vi "编辑控件.vi"(11 "控件类型":string) -> ()   [LabVIEW 2018]
panel:
  in  "图片路径":path
  in  "修改":bool
  in  "删除":bool
  in  "增加":bool
  in  "控件列表":i32(listbox)
  out "图片预览":picture
  in  "程序文本":string
  in  "关键字":string
  in  "控件名称":string
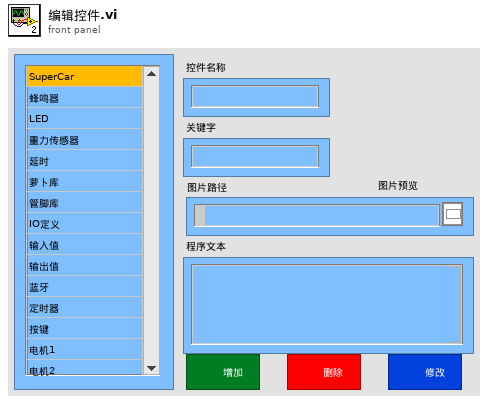
[diagram p1: front panel]
types:
  T1 = typedef "imagedata.ctl" = cluster{"image type":i32, "image depth":i32, "image":u8[], "mask":u8[], "colors":u32[], "Rectangle":cluster{"left":i16, "top":i16, "right":i16, "bottom":i16}}
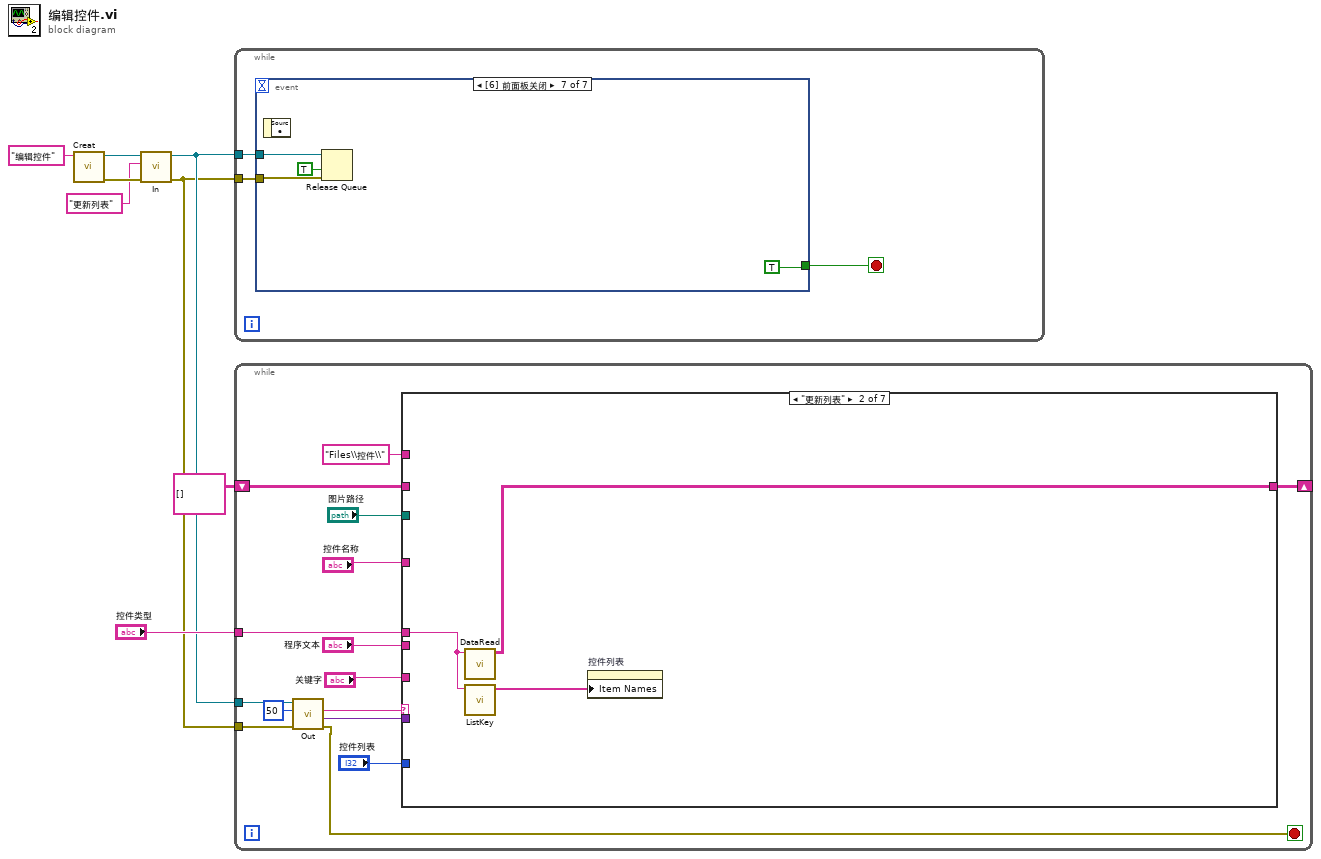
[diagram p0: block diagram]
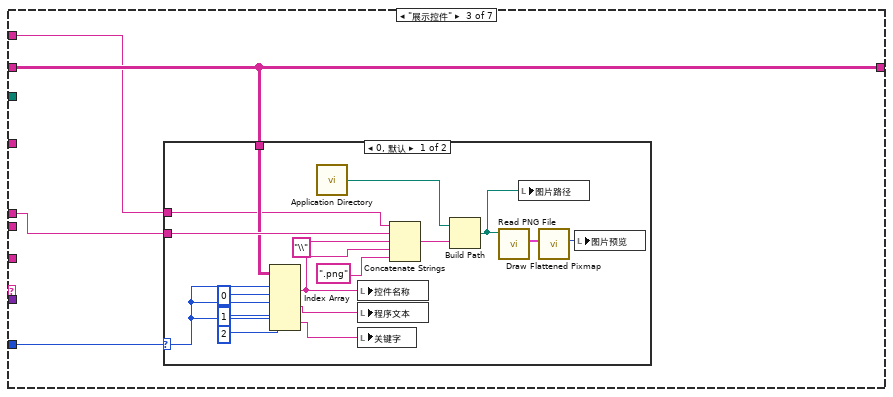
[diagram p3: hidden frame]
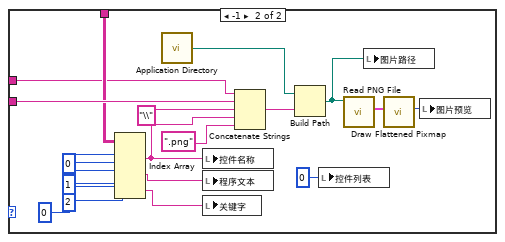
[diagram p4: hidden frame]
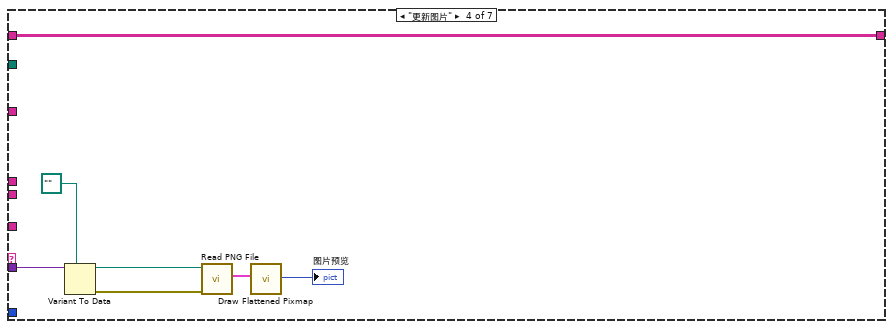
[diagram p5: hidden frame]
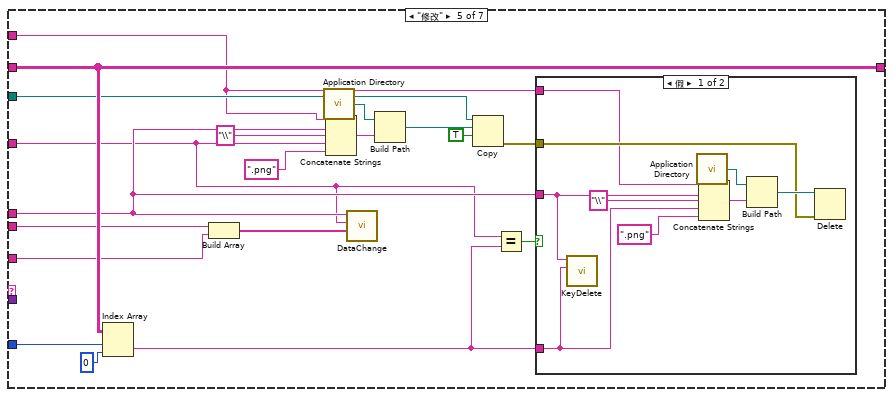
[diagram p6: hidden frame]
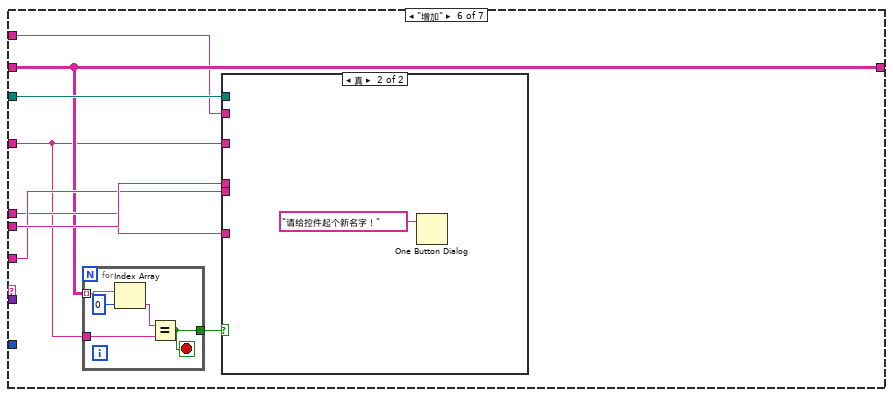
[diagram p8: hidden frame]
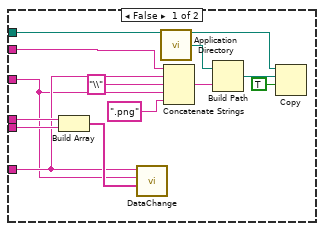
[diagram p9: hidden frame]
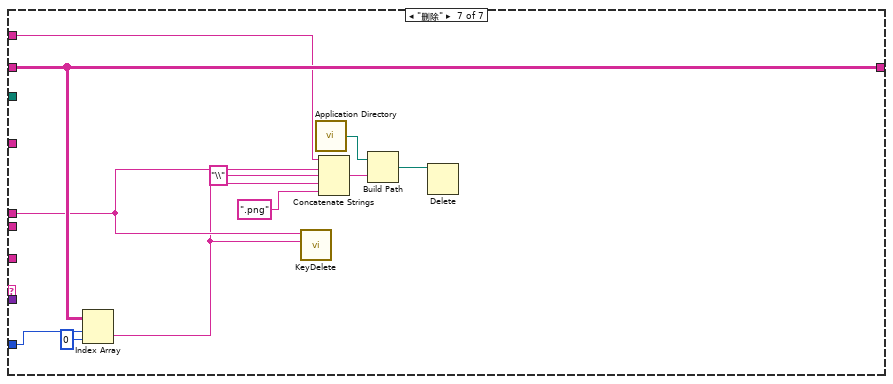
[diagram p10: hidden frame]
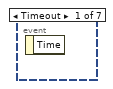
[diagram p11: hidden frame]
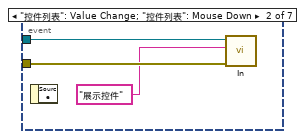
[diagram p12: hidden frame]
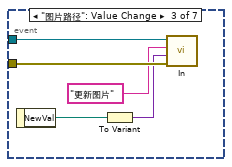
[diagram p13: hidden frame]
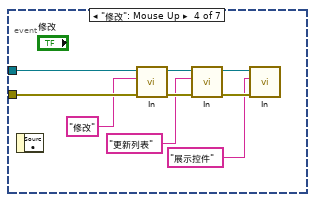
[diagram p14: hidden frame]
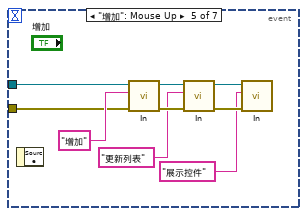
[diagram p15: hidden frame]
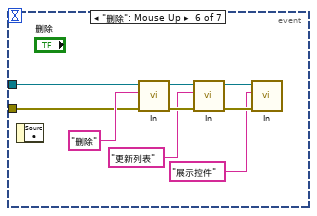
[diagram p16: hidden frame]
diagram:
  n1 = call "Creat.vi"("名称"="编辑控件") -> ("错误输出"=w2:errorcluster, "队列输出"=w5:refnum<queue>)  [unwired: 9 in]
  n2 = call "In.vi"("错误输入"=w2, "指令"="更新列表", "队列"=w5) -> ("错误输出"=w3:errorcluster, "队列输出"=w4:refnum<queue>)  [unwired: 7 in]
  n3 = while {
    tunnel: w4 -> [w11]
    tunnel: w3 -> [w10]
    stop <- w9 stop-if-true
    n4 = event shown="[6] 前面板关闭" {
      selector: _ -> [_ _ _ _ _ _ _]
      dyn-events: _ -> [_ _ _ _ _ _ _]
      timeout: _ -> [_ _ _ _ _ _ _]
      tunnel: w11 -> [_ w14 w19 w28 w30 w39 w49]
      tunnel: w10 -> [_ w13 w18 w27 w29 w38 w48]
      tunnel: [_ _ _ _ _ _ TRUE] -> w9
      event Timeout {
        n5 = event-data() -> ()  [unwired: 1 in, 1 out]
      }
      event "控件列表": Value Change; "控件列表": Mouse Down {
        n6 = event-data() -> ()  [unwired: 1 in, 1 out]
        n7 = call "In.vi"("错误输入"=w13, "指令"="展示控件", "队列"=w14) -> ()  [unwired: 7 in, 2 out]
      }
      event "图片路径": Value Change {
        n8 = event-data() -> ("NewVal"=w17:path)  [unwired: 1 in]
        n9 = To Variant(anything=w17) -> (Variant=w15:variant)
        n10 = call "In.vi"("错误输入"=w18, "数据"=w15, "指令"="更新图片", "队列"=w19) -> ()  [unwired: 6 in, 2 out]
      }
      event "修改": Mouse Up {
        n11 = event-data() -> ()  [unwired: 1 in, 1 out]
        n12 = call "In.vi"("错误输入"=w27, "指令"="修改", "队列"=w28) -> ("错误输出"=w24:errorcluster, "队列输出"=w25:refnum<queue>)  [unwired: 7 in]
        n13 = call "In.vi"("错误输入"=w24, "指令"="更新列表", "队列"=w25) -> ("错误输出"=w22:errorcluster, "队列输出"=w23:refnum<queue>)  [unwired: 7 in]
        n14 = call "In.vi"("错误输入"=w22, "指令"="展示控件", "队列"=w23) -> ()  [unwired: 7 in, 2 out]
      }
      event "增加": Mouse Up {
        n15 = event-data() -> ()  [unwired: 1 in, 1 out]
        n16 = call "In.vi"("错误输入"=w29, "指令"="增加", "队列"=w30) -> ("错误输出"=w35:errorcluster, "队列输出"=w36:refnum<queue>)  [unwired: 7 in]
        n17 = call "In.vi"("错误输入"=w35, "指令"="更新列表", "队列"=w36) -> ("错误输出"=w33:errorcluster, "队列输出"=w34:refnum<queue>)  [unwired: 7 in]
        n18 = call "In.vi"("错误输入"=w33, "指令"="展示控件", "队列"=w34) -> ()  [unwired: 7 in, 2 out]
      }
      event "删除": Mouse Up {
        n19 = event-data() -> ()  [unwired: 1 in, 1 out]
        n20 = call "In.vi"("错误输入"=w38, "指令"="删除", "队列"=w39) -> ("错误输出"=w44:errorcluster, "队列输出"=w45:refnum<queue>)  [unwired: 7 in]
        n21 = call "In.vi"("错误输入"=w44, "指令"="更新列表", "队列"=w45) -> ("错误输出"=w42:errorcluster, "队列输出"=w43:refnum<queue>)  [unwired: 7 in]
        n22 = call "In.vi"("错误输入"=w42, "指令"="展示控件", "队列"=w43) -> ()  [unwired: 7 in, 2 out]
      }
      event Panel Close {
        n23 = event-data() -> ()  [unwired: 1 in, 1 out]
        n24 = Release Queue(queue=w49, force destroy? (F)=TRUE ("强制销毁？(F)"), error in (no error)=w48) -> ()  [unwired: 3 out]
      }
    }
  }
  n25 = while {
    tunnel: w4 -> [w57]
    tunnel: w3 -> [w56]
    shift-right: [w65] -> _
    shift-left: string[][] [] ("数据") -> [w64]
    tunnel: "控件类型" -> [w63]
    stop <- w53 stop-if-true
    n26 = call "Out.vi"("错误输入"=w56, "超时毫秒(-1)"=50, "队列"=w57) -> ("错误输出"=w53:errorcluster, "数据"=w54:variant, "指令"=w55:string)  [unwired: 5 in, 1 out]
    n27 = case shown="\"更新列表\"" w55 {
      tunnel: w54 -> [_ _ _ w110 _ _ _]
      tunnel: [w66 w68 w72 w114 w127 w147 w181] -> w65
      tunnel: w64 -> [w66 _ w72 w114 w127 w147 w181]
      tunnel: w63 -> [_ w69 w73 _ w121 w149 w174]
      tunnel: "控件名称" -> [_ _ _ _ w118 w146 _]
      tunnel: "程序文本" -> [_ _ _ _ w125 w151 _]
      tunnel: "关键字" -> [_ _ _ _ w124 w150 _]
      tunnel: "控件列表" -> [_ _ w71 _ w123 _ w180]
      tunnel: "图片路径" -> [_ _ _ _ w122 w148 _]
      tunnel: "Files\\控件\\" ("名称或相对路径") -> [_ _ w70 _ w116 w144 w171]
      frame "null", Default {
      }
      frame "更新列表" {
        n28 = call "DataRead.vi"("段名"=w69) -> ("数据"=w68:string[][])  [unwired: 10 in]
        n29 = call "ListKey.vi"("section"=w69) -> ("keys"=w67:string[])  [unwired: 10 in]
        n30 = property on="控件列表" class="LstBox (严格)"("Item Names"=w67) -> ()  [unwired: 2 in, 2 out]
      }
      frame "展示控件" {
        n31 = case shown="0, 默认" w71 {
          selector: w71 -> [w75 _]
          tunnel: w73 -> [w78 w96]
          tunnel: w72 -> [w76 w94]
          tunnel: w70 -> [w74 w91]
          frame 0, Default {
            n32 = Index Array(array=w76, index (row) #1=w75, index (col) #1=0 ("禁用的索引 (列)"), index (row) #2=w75, index (col) #2=1 ("禁用的索引 (列)"), index (row) #3=w75, index (col) #3=2 ("禁用的索引 (列)")) -> (element #1=w77:string, element #2=w89:string, element #3=w90:string)
            n33 = call <vilib>:"Application Directory.vi"() -> ("Application Directory"=w79:path)
            n34 = local write "控件名称"(w77) -> ()
            n35 = local write "程序文本"(w89) -> ()
            n36 = local write "关键字"(w90) -> ()
            n37 = Concatenate Strings(w74, w78, "\\" ("字符串"), w77, ".png" ("字符串")) -> (w80:string)
            n38 = Build Path(base path=w79, name or relative path=w80) -> (appended path=w85:path)
            n39 = call <vilib>:"Read PNG File.vi"("path to PNG file"=w85) -> ("image data"=w83:T1)  [unwired: 8 in, 2 out]
            n40 = local write "图片路径"(w85) -> ()
            n41 = call <vilib>:"Draw Flattened Pixmap.vi"("image data"=w83) -> ("new picture"=w84:picture)  [unwired: 8 in]
            n42 = local write "图片预览"(w84) -> ()
          }
          frame -1 {
            w93 = 0 ("禁用的索引 (列)")
            n43 = Index Array(array=w94, index (row) #1=w93, index (col) #1=0 ("禁用的索引 (列)"), index (row) #2=w93, index (col) #2=1 ("禁用的索引 (列)"), index (row) #3=w93, index (col) #3=2 ("禁用的索引 (列)")) -> (element #1=w95:string, element #2=w107:string, element #3=w108:string)
            n44 = call <vilib>:"Application Directory.vi"() -> ("Application Directory"=w97:path)
            n45 = local write "控件名称"(w95) -> ()
            n46 = local write "程序文本"(w107) -> ()
            n47 = local write "关键字"(w108) -> ()
            n48 = Concatenate Strings(w91, w96, "\\" ("字符串"), w95, ".png" ("字符串")) -> (w98:string)
            n49 = Build Path(base path=w97, name or relative path=w98) -> (appended path=w103:path)
            n50 = local write "控件列表"(0 ("控件列表")) -> ()
            n51 = call <vilib>:"Read PNG File.vi"("path to PNG file"=w103) -> ("image data"=w101:T1)  [unwired: 8 in, 2 out]
            n52 = local write "图片路径"(w103) -> ()
            n53 = call <vilib>:"Draw Flattened Pixmap.vi"("image data"=w101) -> ("new picture"=w102:picture)  [unwired: 8 in]
            n54 = local write "图片预览"(w102) -> ()
          }
        }
      }
      frame "更新图片" {
        n55 = Variant To Data(type=path "" ("类型"), Variant=w110) -> (data=w113:path, error out=w109:errorcluster)  [unwired: 1 in]
        n56 = call <vilib>:"Read PNG File.vi"("error in (no error)"=w109, "path to PNG file"=w113) -> ("image data"=w115:T1)  [unwired: 7 in, 2 out]
        n57 = call <vilib>:"Draw Flattened Pixmap.vi"("image data"=w115) -> ("new picture"=→"图片预览":picture)  [unwired: 8 in]
      }
      frame "修改" {
        n58 = Index Array(array=w127, index (row)=w123, index (col)=0 ("禁用的索引 (列)")) -> (element=w117:string)
        n59 = Build Array(w125, w124) -> (w128:string[])
        n60 = call <vilib>:"Application Directory.vi"() -> ("Application Directory"=w131:path)
        n61 = Concatenate Strings(w116, w121, "\\" ("字符串"), w118, ".png" ("字符串")) -> (w132:string)
        n62 = call "DataChange.vi"("值"=w128, "键名"=w118, "段名"=w121) -> ()  [unwired: 9 in]
        n63 = Build Path(base path=w131, name or relative path=w132) -> (appended path=w133:path)
        n64 = Copy(9:TRUE ("覆盖(F)"), 10:w133, 11:w122) -> (0:w120:errorcluster)  [unwired: 2 in, 2 out]
        n65 = Equal?(x=w118, y=w117) -> (x = y?=w119:bool)
        n66 = case shown="假" w119 {
          tunnel: w121 -> [w137 _]
          tunnel: w117 -> [w136 _]
          tunnel: w120 -> [w138 _]
          tunnel: w116 -> [w135 _]
          frame False {
            n67 = call "KeyDelete.vi"("键名"=w136, "段名"=w137) -> ()  [unwired: 10 in]
            n68 = call <vilib>:"Application Directory.vi"() -> ("Application Directory"=w141:path)
            n69 = Concatenate Strings(w135, w137, "\\" ("字符串"), w136, ".png" ("字符串")) -> (w140:string)
            n70 = Build Path(base path=w141, name or relative path=w140) -> (appended path=w139:path)
            n71 = Delete(path (use dialog)=w139, error in=w138) -> ()  [unwired: 3 in, 3 out]
          }
          frame True {
          }
        }
      }
      frame "增加" {
        n72 = for {
          tunnel: w147 -> [w156] mode=indexing
          tunnel: w146 -> [w153]
          tunnel: [w152] -> w145
          stop <- w152 stop-if-true
          n73 = Index Array(array=w156, index=0 ("索引")) -> (element=w154:string)
          n74 = Equal?(x=w154, y=w153) -> (x = y?=w152:bool)
        }
        n75 = case shown="真" w145 {
          tunnel: w151 -> [w169 _]
          tunnel: w150 -> [w168 _]
          tunnel: w149 -> [w162 _]
          tunnel: w146 -> [w158 _]
          tunnel: w148 -> [w160 _]
          tunnel: w144 -> [w157 _]
          frame False {
            n76 = Build Array(w169, w168) -> (w167:string[])
            n77 = call "DataChange.vi"("值"=w167, "键名"=w158, "段名"=w162) -> ()  [unwired: 9 in]
            n78 = call <vilib>:"Application Directory.vi"() -> ("Application Directory"=w165:path)
            n79 = Concatenate Strings(w157, w162, "\\" ("字符串"), w158, ".png" ("字符串")) -> (w166:string)
            n80 = Build Path(base path=w165, name or relative path=w166) -> (appended path=w161:path)
            n81 = Copy(9:TRUE ("覆盖(F)"), 10:w161, 11:w160) -> ()  [unwired: 2 in, 3 out]
          }
          frame True {
            n82 = One Button Dialog(message="请给控件起个新名字！" ("消息")) -> ()  [unwired: 1 in, 1 out]
          }
        }
      }
      frame "删除" {
        n83 = Index Array(array=w181, index (row)=w180, index (col)=0 ("禁用的索引 (列)")) -> (element=w172:string)
        n84 = call "KeyDelete.vi"("键名"=w172, "段名"=w174) -> ()  [unwired: 10 in]
        n85 = call <vilib>:"Application Directory.vi"() -> ("Application Directory"=w177:path)
        n86 = Concatenate Strings(w171, w174, "\\" ("字符串"), w172, ".png" ("字符串")) -> (w178:string)
        n87 = Build Path(base path=w177, name or relative path=w178) -> (appended path=w173:path)
        n88 = Delete(path (use dialog)=w173) -> ()  [unwired: 4 in, 3 out]
      }
    }
  }
